vi "Read 2.vi"(8 "error in (no error)":errorcluster, 11 "State in":T1={"State"=enum."Idle", "Start Time"=timestamp(0 s since 1904-01-01), "Configuration"={"Cycle Period"=0.0, "Mettler"={"VISA resource name"="", "Simulated?"=FALSE}, "Scale Type"=""}, "Current Time"=timestamp(0 s since 1904-01-01), "First Iteration"=FALSE, "Data"={"Scale Read(g)"=0.0}, "Process Name"="", "Log Started"=FALSE}) -> (0 "error out":errorcluster, 3 "State out":T1={"State"=enum."Idle", "Start Time"=timestamp(0 s since 1904-01-01), "Configuration"={"Cycle Period"=0.0, "Mettler"={"VISA resource name"="", "Simulated?"=FALSE}, "Scale Type"=""}, "Current Time"=timestamp(0 s since 1904-01-01), "First Iteration"=FALSE, "Data"={"Scale Read(g)"=0.0}, "Process Name"="", "Log Started"=FALSE})   [LabVIEW 2021, in "Mettler Toledo.lvlib"]
uses:
  Mettler Toledo.lvlib
  Scale Module Folder/Measure Instrument/State Cluster.ctl
  Scale Module Folder/Measure Instrument/State Enum.ctl
  Scale Module Folder/Feed Module/Controls/Scale Module Settings Cluster.ctl
  Controls/Settings Cluster.ctl
  Tag VIs/Tag FGV Operation Enum.ctl
  Scale Module Folder/Measure Instrument/Scale Module Engine.lvlib
  Shared Variables/Dynamic Shared Variables.lvlib
  Scale Module Folder/Scale Module.lvlib
panel:
  # "Scale Settings"
  # "Scale Settings"
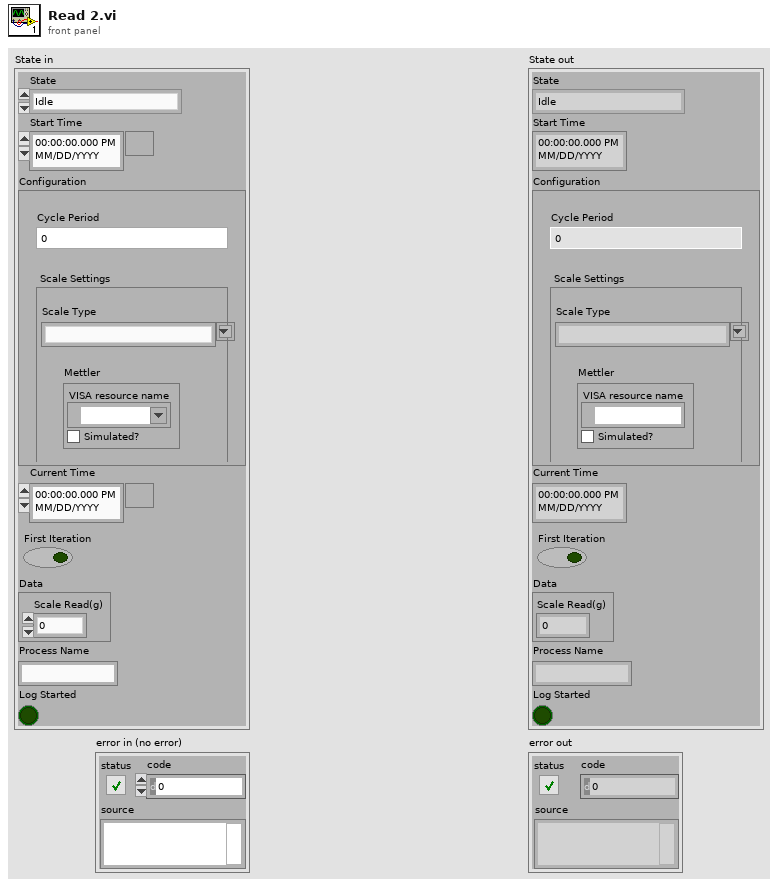
[diagram p1: front panel]
types:
  T1 = typedef "Scale Module.lvlib/Scale Module Engine.lvlib/State Cluster.ctl" = cluster{"State":T2, "Start Time":timestamp, "Configuration":T3, "Current Time":timestamp, "First Iteration":bool, "Data":cluster{"Scale Read(g)":dbl}, "Process Name":string, "Log Started":bool}
  T2 = typedef "Scale Module.lvlib/Scale Module Engine.lvlib/State Enum.ctl" = enum16{"Measuring", "Idle"}
  T3 = typedef "Scale Module.lvlib/Scale Module Settings Cluster.ctl" = cluster{"Cycle Period":dbl, "Mettler":T4, "Scale Type":string}
  T4 = typedef "Mettler Toledo.lvlib/Settings Cluster.ctl" = cluster{"VISA resource name":refnum<visa-resource-name>, "Simulated?":bool}
  T5 = typedef "Tag FGV Operation Enum.ctl" = enum16{"Init", "Set Notification Queue", "Create Tag", "Commit", "Write Tag (Numeric)", "Write Tag (Boolean)", "Read All Tags", "Read One Tag", "Delete Tag Category", "Set Alarm Parameters (Numeric)", "Set Alarm Parameters (Boolean)", "Enable All Alarms", "Disable All Alarms", "Delete All Tags", "Read Alarms", "Ack Alarm", "Read Alarm Parameters (Numeric)", "Read Alarm Parameters (Boolean)"}
  T6 = cluster{"Scale Tag":string, "Output Device Tag":string}
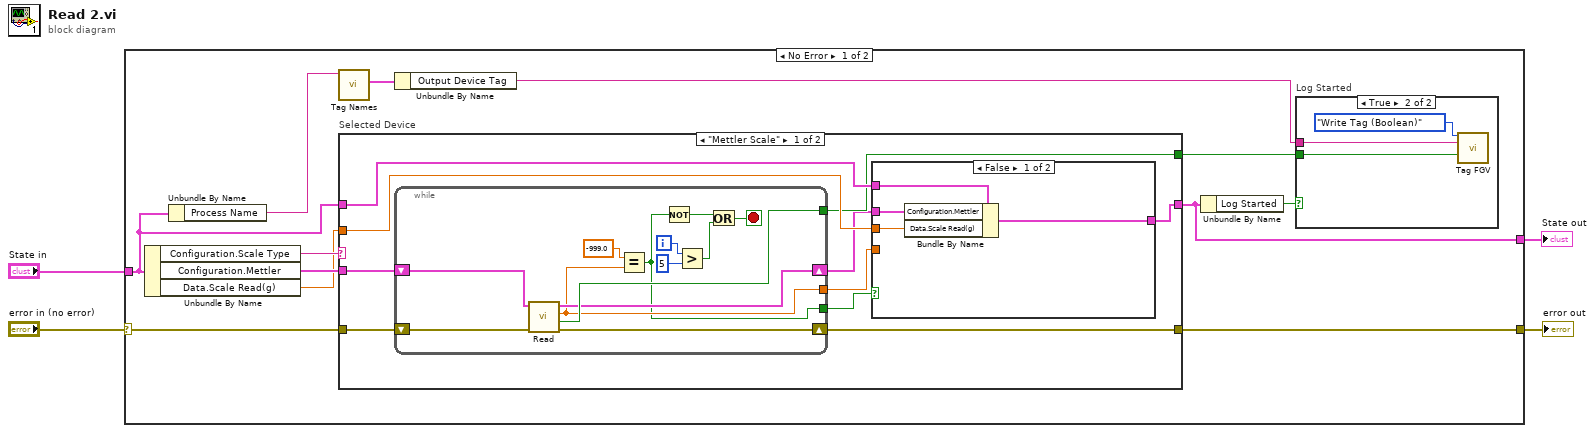
[diagram p0: block diagram]
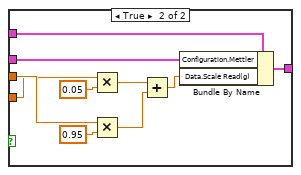
[diagram p3: hidden frame]
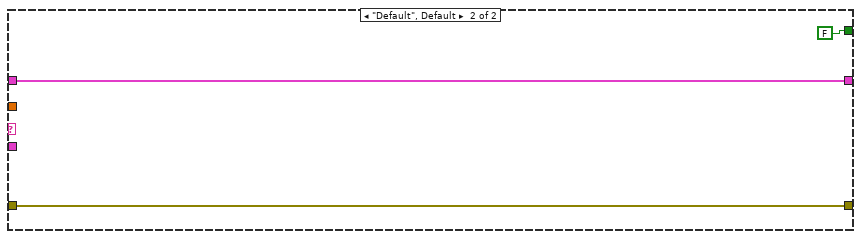
[diagram p4: hidden frame]
diagram:
  n1 = case shown="No Error" "error in (no error)" {
    selector: "error in (no error)" -> [w14 w61]
    tunnel: [w13 w61] -> w1
    tunnel: "State in" -> [w10 w60]
    tunnel: [w6 w60] -> w2
    frame No Error {
      n2 = Unbundle By Name(w10) -> ("Configuration.Scale Type"=w16:string, "Configuration.Mettler"=w15:T4, "Data.Scale Read(g)"=w12:dbl)
      n3 = Unbundle By Name(w10) -> ("Process Name"=w9:string)
      n4 = call "Tag Names.vi"("Process Name"=w9) -> ("Scale Tags"=w8:T6)  [unwired: 8 in, 2 out]
      n5 = case "Selected Device" shown="\"Mettler Scale\"" w16 {
        tunnel: w10 -> [w27 w59]
        tunnel: [w26 w59] -> w6
        tunnel: w15 -> [w28 _]
        tunnel: w14 -> [w29 w58]
        tunnel: [w25 w58] -> w13
        tunnel: w12 -> [w24 _]
        tunnel: [w23 FALSE ("Connection Error")] -> w11
        frame "Mettler Scale" {
          n6 = while {
            tunnel: [w39] -> w23
            tunnel: [w37] -> w21
            tunnel: [w35] -> w20
            shift-right: [w40] -> w25
            shift-left: w29 -> [w42]
            shift-right: [w38] -> w22
            shift-left: w28 -> [w41]
            i -> [w32]
            stop <- w33 stop-if-true
            n7 = call "Read.vi"("error in (no error)"=w42, "Mettler Settings in"=w41) -> ("error out"=w40:errorcluster, "Connection Error"=w39:bool, "mass (g)"=w37:dbl, "Mettler Settings out"=w38:T4)  [unwired: 6 in]
            n8 = Equal?(x=-999.0, y=w37) -> (x = y?=w35:bool)
            n9 = Not(x=w35) -> (.not. x?=w34:bool)
            n10 = Greater?(x=w32, y=5) -> (0:w30:bool)
            n11 = Or(x=w34, y=w30) -> (x .or. y?=w33:bool)
          }
          n12 = case shown="False" w20 {
            tunnel: w27 -> [w43 w56]
            tunnel: [w44 w55] -> w26
            tunnel: w24 -> [w45 w54]
            tunnel: w22 -> [w46 w53]
            tunnel: w21 -> [_ w52]
            frame False {
              n13 = Bundle By Name(cluster=w43, "Configuration.Mettler"=w46, "Data.Scale Read(g)"=w45) -> (w44:T1)
            }
            frame True {
              n14 = Multiply(x=w52, y=0.05) -> (x*y=w48:dbl)
              n15 = Multiply(x=w54, y=0.95) -> (x*y=w51:dbl)
              n16 = Add(x=w48, y=w51) -> (x+y=w47:dbl)
              n17 = Bundle By Name(cluster=w56, "Configuration.Mettler"=w53, "Data.Scale Read(g)"=w47) -> (w55:T1)
            }
          }
        }
        frame "Default", Default {
        }
      }
      n18 = Unbundle By Name(w8) -> ("Output Device Tag"=w7:string)
      n19 = Unbundle By Name(w6) -> ("Log Started"=w5:bool)
      n20 = case "Log Started" shown="True" w5 {
        tunnel: w11 -> [_ w17]
        tunnel: w7 -> [_ w18]
        frame False {
        }
        frame True {
          n21 = call "Tag FGV.vi"("Operation"=Tag_FGV_Operation_Enum."Write Tag (Boolean)", "Tag Name"=w18, "Data"=w17) -> ()  [unwired: 5 in, 8 out]
        }
      }
    }
    frame Error {
    }
  }
  "error out" <- w1
  "State out" <- w2
